vi "Volt Reader Trigger13.vi"() -> ()   [LabVIEW 2014]
uses:
  Enum State Machine Typedef.ctl
  <vilib>/Utility/error.llb/DialogType.ctl
  <vilib>/_DAQmxBase/Internals/DAQmxBase Create Channel (AI-Voltage-Basic).vi
  <vilib>/_DAQmxBase/Internals/DAQmxBase Timing (Sample Clock).vi
  <vilib>/measure/mamon.llb/Trigger Detection for 1 Channel.vi
  <vilib>/_DAQmxBase/Internals/DAQmxBase Read (Analog 2D DBL NChan NSamp).vi
  <vilib>/measure/NI_MAPro.lvlib
  <vilib>/Analysis/NI_AAL_SigProc.lvlib
panel:
  in  "hysteresis":dbl(knob) scale=0.0..10.0
  in  "Center":bool
  in  "Offset (percent of buffer)":dbl(knob) scale=-50.0..50.0
  out "State":T1
  out "Waveform Graph":waveform(dbl)(graph)
  in  "Buffer (Seconds)":dbl
  out "Threshold":dbl
  in  "units":i32(ring)=10348 items=["Volts"=10348, "From Custom Scale"=10065]
  in  "stop":bool
  in  "physical channels":tag
  in  "maximum value":dbl=5.0 format="%0.2f"
  in  "minimum value":dbl=-5.0 format="%0.2f"
  in  "rate":i32=1000 caption="Sample Rate"
  # "The inputs above MUST BE\nPreset before running"
  # "NOTE: Just change the Y axis value"
  # "Make Sure that Buffer does not equal 0"
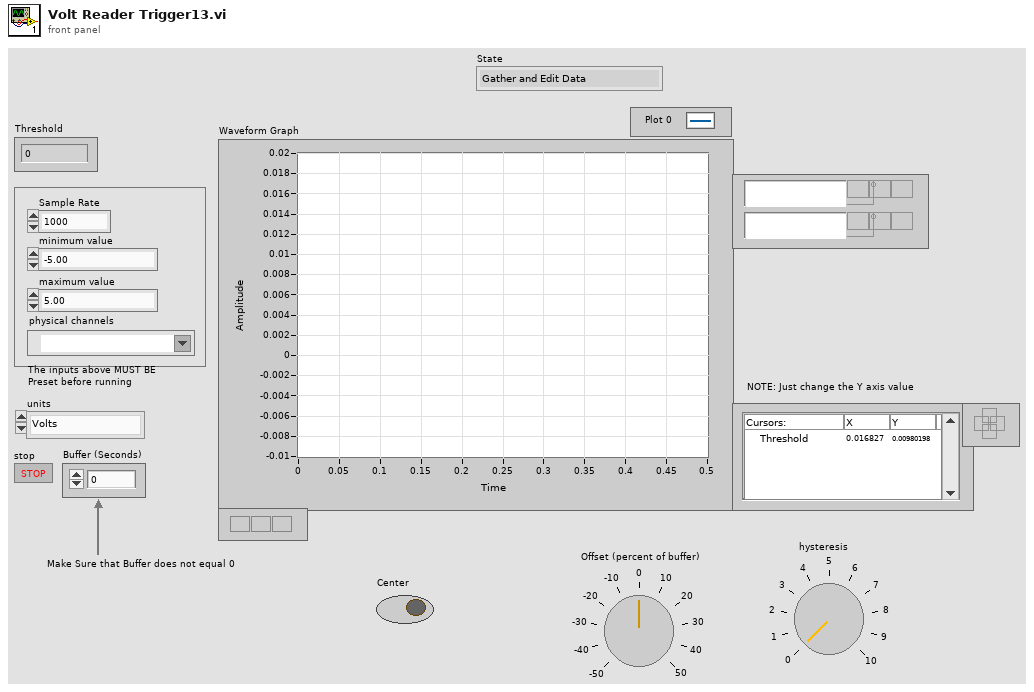
[diagram p1: front panel]
types:
  T1 = typedef "Enum State Machine Typedef.ctl" = enum16{"Gather and Edit Data", "Trigger Occured", "Just Displayed"}
  T2 = typedef "DialogType.ctl" = u16
  T3 = typedef "LVCursorListTypeDef.ctl" = cluster{"Name":string, "Color":u32, "Style":u8, "Point Style":u8, "Name Visible":bool, "Allow Drag":bool, "Cursor Mode":u32, "Plot":i32, "Index":i32, "Position":cluster{"X":dbl, "Y":dbl}, "X Scale":u32, "Y Scale":u32, "Watch Plots":i32[], "Watch All Plots":bool, "Plot Area":i32, "Label Offset":cluster{"X":dbl, "Y":dbl}}[]
  T4 = cluster{"Name":string, "Color":u32, "Style":u8, "Point Style":u8, "Name Visible":bool, "Allow Drag":bool, "Cursor Mode":u32, "Plot":i32, "Index":i32, "Position":cluster{"X":dbl, "Y":dbl}, "X Scale":u32, "Y Scale":u32, "Watch Plots":i32[], "Watch All Plots":bool, "Plot Area":i32, "Label Offset":cluster{"X":dbl, "Y":dbl}}
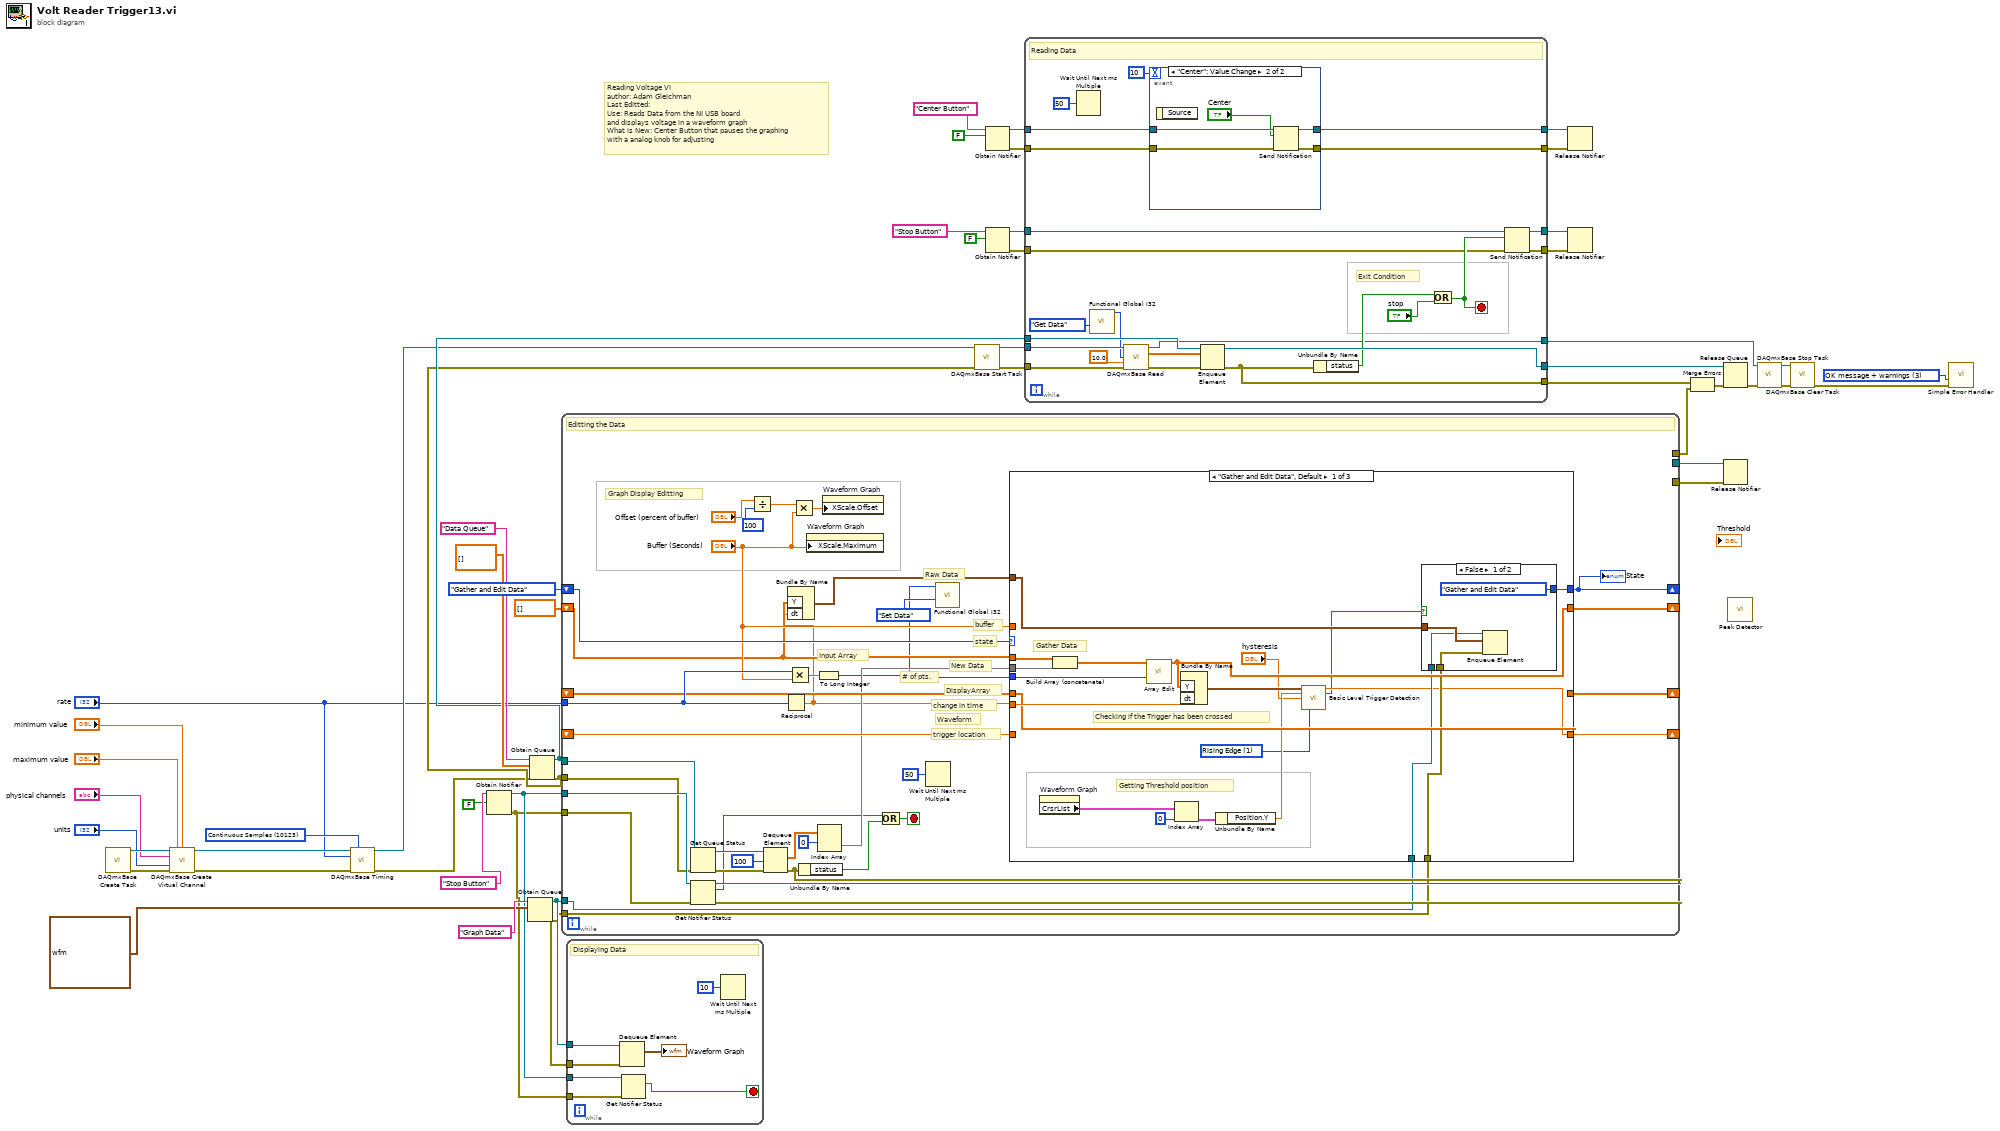
[diagram p0: block diagram]
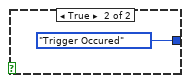
[diagram p2: hidden frame]
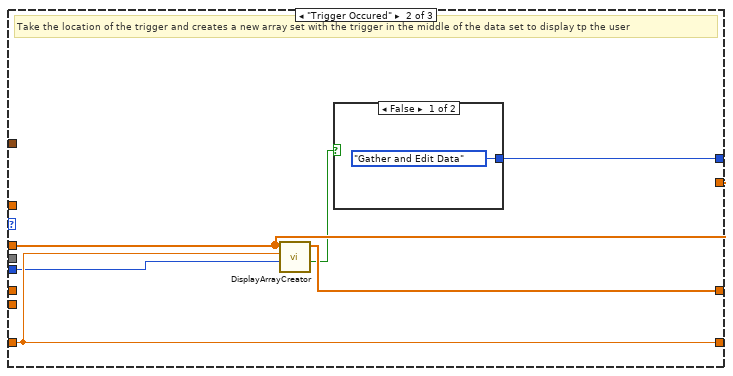
[diagram p3: hidden frame]
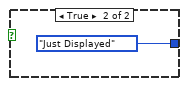
[diagram p4: hidden frame]
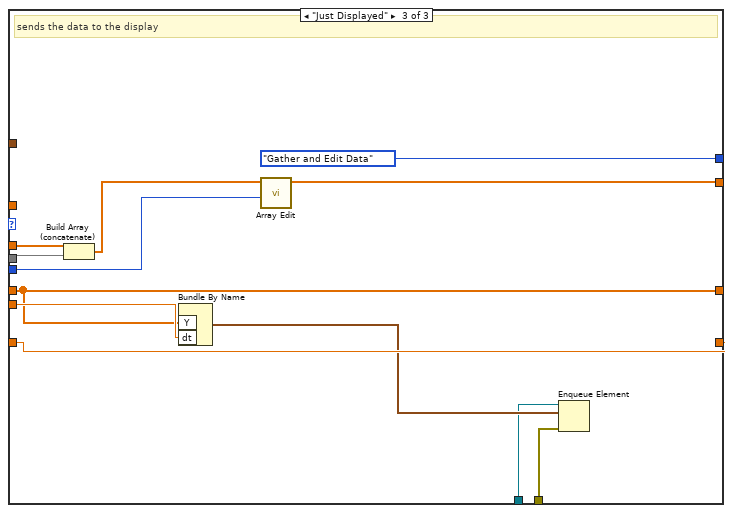
[diagram p5: hidden frame]
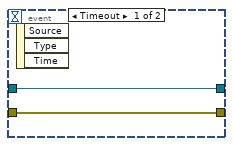
[diagram p6: hidden frame]
diagram:
  w29 = 10123 items=["Finite Samples"=10178, "Continuous Samples"=10123, "Hardware Timed Single Point"=12522] ("sample mode")
  w31 = T2 3 items=["no dialog", "OK message", "continue or stop message", "OK message + warnings", "continue/stop + warnings"] ("type of dialog (OK msg:1)")
  # "Reading Voltage VI\nauthor: Adam Gleichman\nLast Editted: \nUse: Reads Data from the NI USB board\nand displays voltage in a waveform graph\nWhat is New: Center Button that pauses the graphing\nwith a analog knob for adjusting"
  n1 = call <vilib>:"DAQmxBase Create Task.vi"() -> ("task out"=w51:refnum<k21>, "error out"=w50:errorcluster)  [unwired: 5 in, 9 out]
  n2 = call-poly <vilib>:"DAQmxBase Create Virtual Channel.vi"("task in"=w51, "maximum value"="maximum value", "minimum value"="minimum value", "physical channels"="physical channels", "units"="units", "error in"=w50) -> ("task out"=w48:refnum<k21>, "error out"=w49:errorcluster)  [unwired: 3 in, 5 out]
  n3 = call-poly <vilib>:"DAQmxBase Timing.vi"("task/channels in"=w48, "sample mode"=w29, "rate"="rate", "error in"=w49) -> ("task out"=w19:refnum<k21>, "error out"=w18:errorcluster)  [unwired: 3 in, 7 out]
  n4 = Obtain Notifier(name (unnamed)="Stop Button", notification data type=FALSE) -> (notifier out=w2:refnum<notifier>, error out=w1:errorcluster)  [unwired: 2 in, 1 out]
  n5 = Obtain Queue(name (unnamed)="Graph Data", element data type=waveform(dbl) {"t0"=timestamp(0 s since 1904-01-01), "dt"=1.0, "Y"=[]} ("Waveform Graph")) -> (queue out=w4:refnum<queue>, error out=w3:errorcluster)  [unwired: 3 in, 1 out]
  n6 = Obtain Queue(name (unnamed)="Data Queue", element data type=dbl[][] [] ("data"), error in (no error)=w18) -> (queue out=w38:refnum<queue>, error out=w37:errorcluster)  [unwired: 2 in, 1 out]
  n7 = while {
    tunnel: w38 -> [w90]
    tunnel: w37 -> [w81]
    tunnel: [w88] -> w36
    tunnel: w2 -> [w86]
    tunnel: w1 -> [w85]
    tunnel: [w84] -> w20
    tunnel: [w83] -> w21
    tunnel: "rate" -> [w77]
    shift-right: [w59] -> _
    shift-left: dbl[] [] -> [w63]
    shift-right: [w58] -> _
    shift-left: Enum_State_Machine_Typedef."Gather and Edit Data" -> [w74]
    shift-right: [w57] -> _
    shift-left: _ -> [w75]
    shift-right: [w73] -> _
    shift-left: _ -> [w72]
    tunnel: w4 -> [w55]
    tunnel: w3 -> [w54]
    stop <- w87 stop-if-true
    # "Raw Data"
    # "state"
    # "Graph Display Editting"
    # "Waveform"
    # "DisplayArray"
    # "trigger location"
    # "change in time"
    # "buffer"
    # "New Data"
    # "Input Array"
    # "# of pts."
    # "Editting the Data"
    n8 = Get Queue Status(queue=w90, error in (no error)=w81) -> (queue out=w82:refnum<queue>, error out=w80:errorcluster)  [unwired: 1 in, 6 out]
    n9 = Get Notifier Status(notifier=w86, error in (no error)=w85) -> (notifier out=w84:refnum<notifier>, current notification=w64:bool, error out=w83:errorcluster)  [unwired: 2 out]
    n10 = Divide(x="Offset (percent of buffer)", y=100) -> (x/y=w67:dbl)
    n11 = Dequeue Element(queue=w82, timeout in ms (-1)=100, error in (no error)=w80) -> (element=w78:dbl[][], error out=w88:errorcluster)  [unwired: 2 out]
    n12 = Reciprocal(x=w77) -> (1/x=w62:dbl)
    n13 = Bundle By Name("Y"=w63, "dt"=w62) -> (w56:waveform(dbl))  [unwired: 1 in]
    n14 = Multiply(x=w77, y="Buffer (Seconds)") -> (x*y=w76:dbl)
    n15 = Multiply(x=w67, y="Buffer (Seconds)") -> (x*y=w66:dbl)
    n16 = Unbundle By Name(w88) -> ("status"=w65:bool)
    n17 = property on="Waveform Graph" class="WFGraph (strict)"("XScale.Maximum"="Buffer (Seconds)") -> ()  [unwired: 2 in, 2 out]
    n18 = To Long Integer(number=w76) -> (32bit integer=w60:i32)
    n19 = Index Array(array=w78, index (row)=0 ("index")) -> (element=w71:dbl[])  [unwired: 1 in]
    n20 = property on="Waveform Graph" class="WFGraph (strict)"("XScale.Offset"=w66) -> ()  [unwired: 2 in, 2 out]
    n21 = Or(x=w64, y=w65) -> (x .or. y?=w87:bool)
    n22 = Wait Until Next ms Multiple(millisecond multiple=u32 50) -> ()  [unwired: 1 out]
    n23 = call "Functional Global I32.vi"("Enum"=enum16{"Set Data", "Get Data"}."Set Data", "Integer In"=w60) -> ()  [unwired: 9 in, 1 out]
    n24 = case shown="\"Gather and Edit Data\", Default" w74 {
      tunnel: w63 -> [w110 w120 w132]
      tunnel: w71 -> [w109 _ w131]
      tunnel: w62 -> [w105 _ w135]
      tunnel: w60 -> [w107 w118 w129]
      tunnel: w75 -> [w100 _ w133]
      tunnel: "Buffer (Seconds)" -> [_ _ _]
      tunnel: [w94 w119 w134] -> w73
      tunnel: w72 -> [_ w119 w134]
      tunnel: [w106 w120 w128] -> w59
      tunnel: [w104 w117 Enum_State_Machine_Typedef."Gather and Edit Data"] -> w58
      tunnel: [w100 w121 w133] -> w57
      tunnel: w56 -> [w99 _ _]
      tunnel: w55 -> [w98 _ w125]
      tunnel: w54 -> [w97 _ w124]
      frame "Gather and Edit Data", Default {
        w92 = u16 1 items=["Falling Edge", "Rising Edge"] ("trigger slope")
        # "Getting Threshold position"
        # "Checking if the Trigger has been crossed"
        # "Gather Data"
        n25 = property on="Waveform Graph" class="WFGraph (strict)"() -> ("CrsrList"=w101:T3)  [unwired: 2 in, 2 out]
        n26 = Build Array (concatenate)(w110, w109) -> (w108:dbl[])
        n27 = call "Array Edit.vi"("Number of Points"=w107, "Y-values"=w108) -> ("Editted Y Values"=w106:dbl[])  [unwired: 9 in]
        n28 = Index Array(array=w101, index=0) -> (element=w103:T4)
        n29 = Bundle By Name("Y"=w106, "dt"=w105) -> (w96:waveform(dbl))  [unwired: 1 in]
        n30 = Unbundle By Name(w103) -> ("Position.Y"=w95:dbl)
        n31 = call-poly <vilib>:"Basic Level Trigger Detection.vi"("signal in"=w96, "level"=w95, "hysteresis"="hysteresis", "trigger slope"=w92) -> ("trigger location"=w94:dbl, "trigger detected?"=w93:bool)  [unwired: 9 in, 1 out]
        n32 = case shown="False" w93 {
          tunnel: [Enum_State_Machine_Typedef."Gather and Edit Data" Enum_State_Machine_Typedef."Trigger Occured"] -> w104
          tunnel: w99 -> [w113 _]
          tunnel: w98 -> [w111 _]
          tunnel: w97 -> [w112 _]
          frame False {
            n33 = Enqueue Element(queue=w111, element=w113, error in (no error)=w112) -> ()  [unwired: 1 in, 3 out]
          }
          frame True {
          }
        }
      }
      frame "Trigger Occured" {
        # "Take the location of the trigger and creates a new array set with the trigger in the middle of the data set to display tp the user"
        n34 = call "DisplayArrayCreator.vi"("Number of Points"=w118, "Location of the Trigger"=w119, "Input Y Values"=w120) -> ("Valid?"=w116:bool, "Output Y Values"=w121:dbl[])  [unwired: 7 in]
        n35 = case shown="False" w116 {
          tunnel: [Enum_State_Machine_Typedef."Gather and Edit Data" Enum_State_Machine_Typedef."Just Displayed"] -> w117
          frame False {
          }
          frame True {
          }
        }
      }
      frame "Just Displayed" {
        # "sends the data to the display"
        n36 = Build Array (concatenate)(w132, w131) -> (w130:dbl[])
        n37 = Bundle By Name("Y"=w133, "dt"=w135) -> (w126:waveform(dbl))  [unwired: 1 in]
        n38 = call "Array Edit.vi"("Number of Points"=w129, "Y-values"=w130) -> ("Editted Y Values"=w128:dbl[])  [unwired: 9 in]
        n39 = Enqueue Element(queue=w125, element=w126, error in (no error)=w124) -> ()  [unwired: 1 in, 3 out]
      }
    }
    "State" <- w58
  }
  n40 = while {
    tunnel: w4 -> [w142]
    tunnel: w3 -> [w141]
    tunnel: w2 -> [w139]
    tunnel: w1 -> [w138]
    stop <- w137 stop-if-true
    # "Displaying Data"
    n41 = Dequeue Element(queue=w142, error in (no error)=w141) -> (element=→"Waveform Graph":waveform(dbl))  [unwired: 1 in, 3 out]
    n42 = Get Notifier Status(notifier=w139, error in (no error)=w138) -> (current notification=w137:bool)  [unwired: 4 out]
    n43 = Wait Until Next ms Multiple(millisecond multiple=u32 10) -> ()  [unwired: 1 out]
  }
  n44 = call <vilib>:"DAQmxBase Start Task.vi"("task/channels in"=w19, "error in"=w37) -> ("task out"=w46:refnum<k21>, "error out"=w47:errorcluster)  [unwired: 12 out]
  n45 = Obtain Notifier(name (unnamed)="Center Button", notification data type=FALSE) -> (notifier out=w12:refnum<notifier>, error out=w11:errorcluster)  [unwired: 2 in, 1 out]
  n46 = Obtain Notifier(name (unnamed)="Stop Button", notification data type=FALSE) -> (notifier out=w25:refnum<notifier>, error out=w24:errorcluster)  [unwired: 2 in, 1 out]
  n47 = while "Data Reading Loop" {
    tunnel: w47 -> [w165]
    tunnel: w46 -> [w166]
    tunnel: w38 -> [w163]
    tunnel: [w160] -> w41
    tunnel: [w158] -> w40
    tunnel: [w156] -> w28
    tunnel: w25 -> [w154]
    tunnel: w24 -> [w153]
    tunnel: [w152] -> w17
    tunnel: [w151] -> w16
    tunnel: w12 -> [w150]
    tunnel: w11 -> [w149]
    tunnel: [w148] -> w8
    tunnel: [w147] -> w7
    stop <- w155 stop-if-true
    # "Exit Condition"
    # "Reading Data"
    n48 = Wait Until Next ms Multiple(millisecond multiple=u32 50) -> ()  [unwired: 1 out]
    n49 = call "Functional Global I32.vi"("Enum"=enum16{"Set Data", "Get Data"}."Get Data") -> ("Integer"=w145:i32)  [unwired: 10 in]
    n50 = call-poly <vilib>:"DAQmxBase Read.vi"("task/channels in"=w166, "number of samples per channel"=w145, "timeout"=10.0, "error in"=w165) -> ("task out"=w156:refnum<k21>, "data"=w161:dbl[][], "error out"=w164:errorcluster)  [unwired: 9 in]
    n51 = event shown="[1] \"Center\": Value Change" {
      selector: _ -> [_ _]
      dyn-events: _ -> [_ _]
      timeout: 10 -> [_ _]
      tunnel: w150 -> [w168 w173]
      tunnel: w149 -> [w167 w172]
      tunnel: [w168 w170] -> w148
      tunnel: [w167 w169] -> w147
      event Timeout {
        n52 = event-data() -> ()  [unwired: 1 in, 3 out]
      }
      event "Center": Value Change {
        n53 = event-data() -> ()  [unwired: 1 in, 1 out]
        n54 = Send Notification(notification="Center", notifier=w173, error in (no error)=w172) -> (notifier out=w170:refnum<notifier>, error out=w169:errorcluster)
      }
    }
    n55 = Enqueue Element(queue=w163, element=w161, error in (no error)=w164) -> (queue out=w160:refnum<queue>, error out=w158:errorcluster)  [unwired: 1 in, 1 out]
    n56 = Unbundle By Name(w158) -> ("status"=w157:bool)
    n57 = Or(x=w157, y="stop") -> (x .or. y?=w155:bool)
    n58 = Send Notification(notification=w155, notifier=w154, error in (no error)=w153) -> (notifier out=w152:refnum<notifier>, error out=w151:errorcluster)
  }
  n59 = Release Notifier(notifier=w8, error in (no error)=w7) -> ()  [unwired: 1 in, 3 out]
  n60 = Release Notifier(notifier=w17, error in (no error)=w16) -> ()  [unwired: 1 in, 3 out]
  n61 = Merge Errors(w40, w36) -> (w39:errorcluster)
  n62 = Release Queue(queue=w41, error in (no error)=w39) -> (error out=w35:errorcluster)  [unwired: 1 in, 2 out]
  n63 = Release Notifier(notifier=w20, error in (no error)=w21) -> ()  [unwired: 1 in, 3 out]
  n64 = call <vilib>:"Peak Detector.vi"() -> ()  [unwired: 7 in, 5 out]
  n65 = call <vilib>:"DAQmxBase Stop Task.vi"("task/channels in"=w28, "error in"=w35) -> ("task out"=w34:refnum<k21>, "error out"=w33:errorcluster)  [unwired: 12 in]
  n66 = call <vilib>:"DAQmxBase Clear Task.vi"("task in"=w34, "error in"=w33) -> ("error out"=w32:errorcluster)  [unwired: 13 in]
  n67 = call <vilib>:"Simple Error Handler.vi"("type of dialog (OK msg:1)"=w31, "error in (no error)"=w32) -> ()  [unwired: 3 in, 5 out]
